vi "SlewRateLimiter_New.vi"(9 "InitialValue":dbl, 11 "RateLimit":dbl) -> (3 "out SLEW_RATE_LIMITER":T1 {"PrevTime" format="%30.5p"; "PrevValue" format="%13.5p"; "RateLimit" format="%13.5p"})   [LabVIEW 2019, in "Trajectory_Library.lvlib"]
doc: "Creates a new SlewRateLimiter data cluster with the given rate limit and initial value.\n\nThis set of functions limits the rate of change of an input value. Useful for implementing voltage, setpoint, and/or output ramps. A slew-rate limit is most appropriate when the quantity being controlled is a velocity or a voltage; when controlling a position, consider using a postion control algoritmn or trapezoid profile instead.\n\nInputs:\n - rateLimit -- The rate-of-change limit, in units per second.\n - initialValue -- The initial value of the input.\n \nOutputs:\n - out Slew Rate Limiter -- The initialized Slew Rate Limiter data cluster"
uses:
  Trajectory_Library.lvlib
  SLEW_RATE_LIMITER.ctl
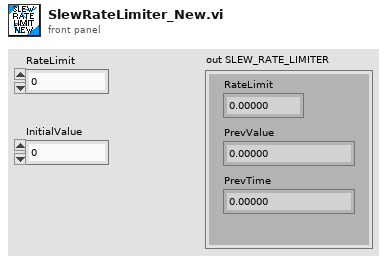
[diagram p1: front panel]
types:
  T1 = typedef "Trajectory_Library.lvlib/SLEW_RATE_LIMITER.ctl" = cluster{"RateLimit":dbl, "PrevValue":dbl, "PrevTime":dbl}
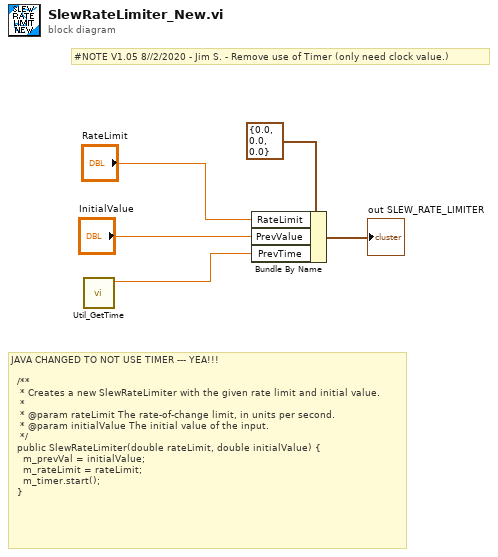
[diagram p0: block diagram]
diagram:
  # "#NOTE V1.05 8//2/2020 - Jim S. - Remove use of Timer (only need clock value.)"
  # "JAVA CHANGED TO NOT USE TIMER --- YEA!!!\n\n  /**\n   * Creates a new SlewRateLimiter with the given rate limit and initial value.\n   *\n   * @param rateLimit The rate-of-change limit, in units per second.\n   * @param initialValue The initial value of the input.\n   */\n  public SlewRateLimiter(double rateLimit, double initialValue) {\n    m_prevVal = initialValue;\n    m_rateLimit = rateLimit;\n    m_timer.start();\n  }"
  n1 = call "Util_GetTime.vi"() -> ("FPGA_Time_Seconds"=w1:dbl)  [unwired: 10 in, 1 out]
  n2 = Bundle By Name(cluster=T1 {"RateLimit"=0.0, "PrevValue"=0.0, "PrevTime"=0.0} ("out SLEW_RATE_LIMITER"), "RateLimit"="RateLimit", "PrevValue"="InitialValue", "PrevTime"=w1) -> (→"out SLEW_RATE_LIMITER":T1)
